vi "PointsDist.vi"(10 "Point2":T1, 11 "Point1":T1) -> (3 "Dist":sgl)   [LabVIEW 2014]
uses:
  TypeDefs/Point2DwSlope.ctl
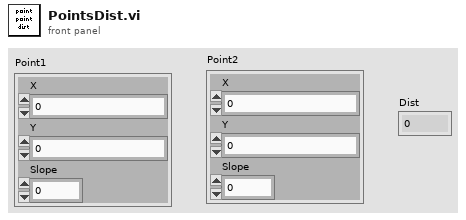
[diagram p1: front panel]
types:
  T1 = typedef "Point2DwSlope.ctl" = cluster{"X":sgl, "Y":sgl, "Slope":dbl}
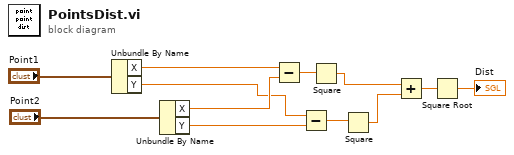
[diagram p0: block diagram]
diagram:
  n1 = Unbundle By Name("Point1") -> ("X"=w10:sgl, "Y"=w7:sgl)
  n2 = Unbundle By Name("Point2") -> ("X"=w9:sgl, "Y"=w8:sgl)
  n3 = Subtract(x=w10, y=w9) -> (x-y=w6:sgl)
  n4 = Subtract(x=w7, y=w8) -> (x-y=w5:sgl)
  n5 = Square(x=w6) -> (x^2=w4:sgl)
  n6 = Square(x=w5) -> (x^2=w3:sgl)
  n7 = Add(x=w4, y=w3) -> (x+y=w2:sgl)
  n8 = Square Root(x=w2) -> (sqrt(x)=→"Dist":sgl)
